vi "Trim String.vi"(3 "String in":string, 4 "Remove White Space":bool=TRUE) -> (5 "Trimmed String":string)   [LabVIEW 2021, in "DataTypes_CIF_U.lvlib"]
doc: "Remove C end of string character (\\0) and trim white space."
uses:
  DataTypes_CIF_U.lvlib
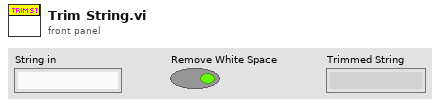
[diagram p1: front panel]
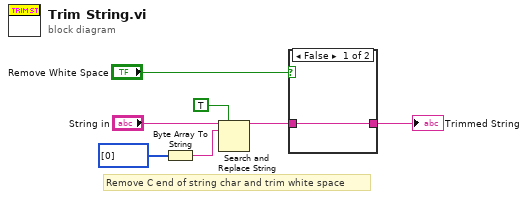
[diagram p0: block diagram]
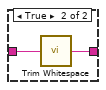
[diagram p2: hidden frame]
diagram:
  # "Remove C end of string char and trim white space"
  n1 = Byte Array To String(unsigned byte array=u8[] [0]) -> (string=w5:string)
  n2 = Search and Replace String(replace all?=TRUE ("replace all? (F)"), input string="String in", search string=w5) -> (result string=w3:string)  [unwired: 5 in, 3 out]
  n3 = case shown="False" "Remove White Space" {
    tunnel: w3 -> [w8 w10]
    tunnel: [w8 w9] -> w2
    frame False {
    }
    frame True {
      n4 = call <vilib>:"Trim Whitespace.vi"("string"=w10) -> ("trimmed string"=w9:string)  [unwired: 1 in]
    }
  }
  "Trimmed String" <- w2
